vi "LVPortSetTempObject.vi"(6 "Nameless Array as Object":bool, 7 "Skip Parent Name":bool=TRUE, 8 "Error in":errorcluster, 9 "ID (-1 = new temp)":i32=-1, 10 "Value":variant, 11 "pID":string) -> (0 "Error out":errorcluster, 2 "Object map":T1[](array[typedef]), 3 "ID (Validated)":i32)   [LabVIEW 2017]
uses:
  Common/ObjectMap/LVPortObjectMapNamepathData.ctl
  Common/ObjectMap/LVPortObjectMapDataTypeEnum.ctl
  Common/ObjectMap/LVPortObjectMapContainerTypeEnum.ctl
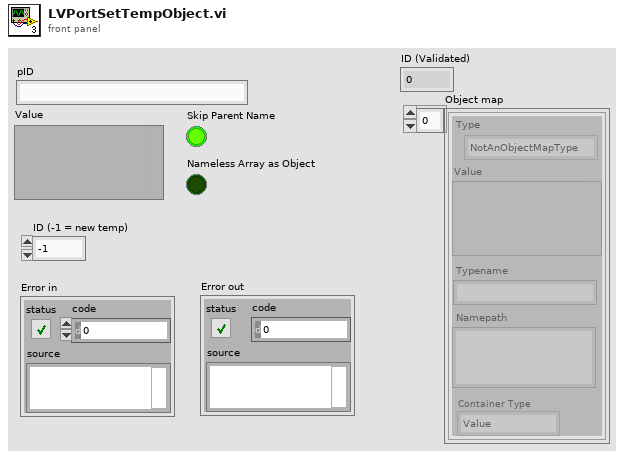
[diagram p1: front panel]
types:
  T1 = typedef "LVPortObjectMapNamepathData.ctl" = cluster{"Type":T2, "Value":variant, "Namepath":string, "Typename":string, "Container Type":T3}
  T2 = typedef "LVPortObjectMapDataTypeEnum.ctl" = enum16{"NotAnObjectMapType", "Real", "Complex", "String", "Boolean"}
  T3 = typedef "LVPortObjectMapContainerTypeEnum.ctl" = enum16{"Value", "Array", "Waveform"}
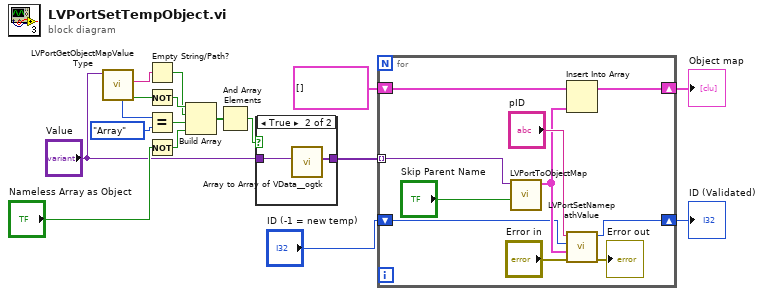
[diagram p0: block diagram]
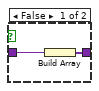
[diagram p2: hidden frame]
diagram:
  n1 = call "LVPortGetObjectMapValueType.vi"("Value"="Value") -> ("IsNumeric"=w9:bool, "Name"=w10:string, "Container Type (Labview Value type)"=w12:T3)  [unwired: 6 in, 2 out]
  n2 = Empty String/Path?(string/path=w10) -> (empty?=w7:bool)
  n3 = Not(x=w9) -> (.not. x?=w8:bool)
  n4 = Equal?(x=w12, y=LVPortObjectMapContainerTypeEnum."Array") -> (x = y?=w6:bool)
  n5 = Not(x="Nameless Array as Object") -> (.not. x?=w5:bool)
  n6 = Build Array(w8, w7, w6, w5) -> (w4:bool[])
  n7 = And Array Elements(Boolean array=w4) -> (logical AND=w3:bool)
  n8 = case shown="True" w3 {
    tunnel: "Value" -> [w19 w21]
    tunnel: [w18 w20] -> w17
    frame False {
      n9 = Build Array(w19) -> (w18:variant[])
    }
    frame True {
      n10 = call <userlib>:"Array to Array of VData__ogtk.vi"("MultiD Array"=w21) -> ("1D Array of Variants"=w20:variant[])  [unwired: 9 in, 1 out]
    }
  }
  n11 = for {
    tunnel: w17 -> [w28] mode=indexing
    shift-right: [w24] -> w15
    shift-left: T1[] [] ("Object map") -> [w26]
    shift-right: [w23] -> w2
    shift-left: "ID (-1 = new temp)" -> [w22]
    n12 = call "LVPortToObjectMap.vi"("Skip Parent Name (t)"="Skip Parent Name", "Value"=w28) -> ("Object map"=w25:T1[])  [unwired: 9 in]
    n13 = Insert Into Array(array=w26, new element=w25) -> (w24:T1[])  [unwired: 1 in]
    n14 = call "LVPortSetNamepathValue.vi"("Error in"="Error in", "ObjectMap"=w25, "Object ID"=w22, "pID"="pID") -> ("Error out"=→"Error out":errorcluster, "Object ID (Validated)"=w23:i32)  [unwired: 5 in, 1 out]
  }
  "Object map" <- w15
  "ID (Validated)" <- w2
